vi "MPB_MAIN.vi"() -> ()   [LabVIEW 2020]
uses:
  controls/step_type.ctl
  controls/step.ctl
  controls/test results.ctl
panel:
  out "test results 2":T1
  out "test results":T1
  in  "Start Test":bool
  in  "Stop Test":bool
  in  "Exit Program":bool
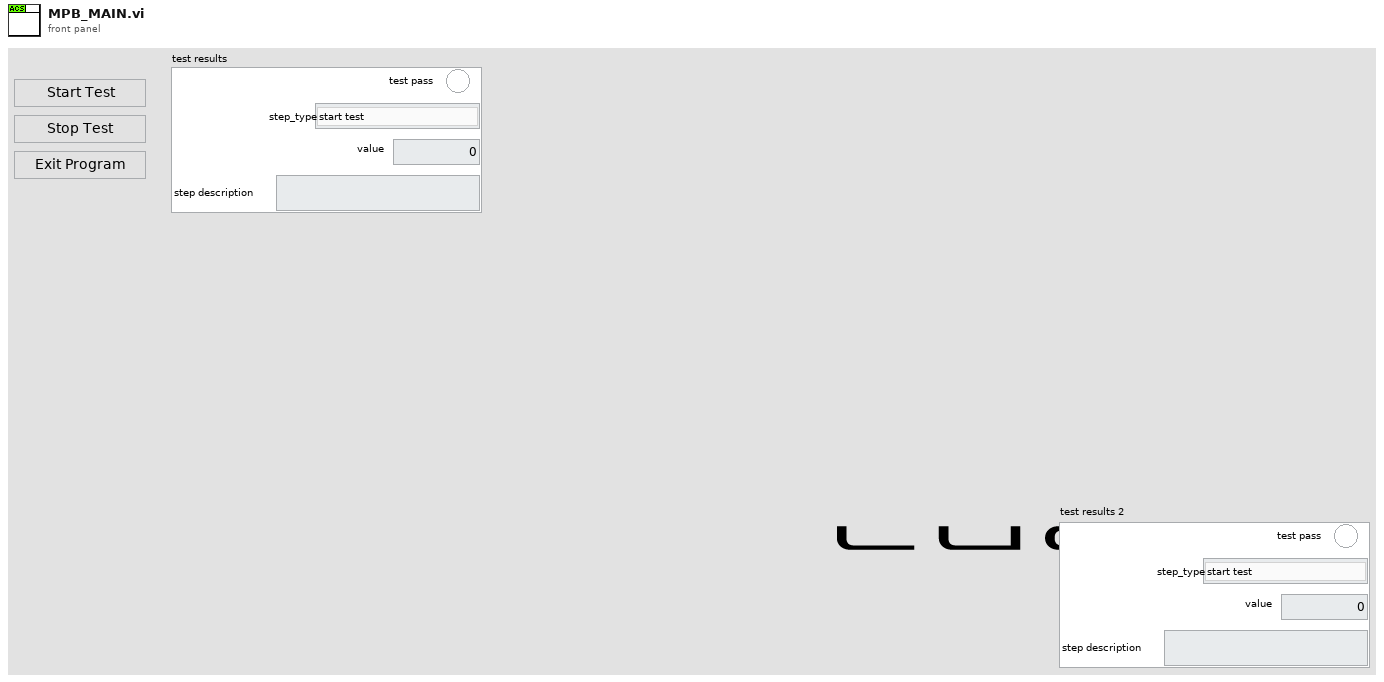
[diagram p1: front panel]
types:
  T1 = typedef "test results.ctl" = cluster{"test pass":bool, "step_type":T2, "value":dbl, "step description":string}
  T2 = typedef "step_type.ctl" = enum16{"start test", "prompt", "sequence#", "12V power supply on_off", "set_hipot_V", "set_hipot_I_limit", "set_hipot_ramping (sec)", "read_hipot_V", "read_hipot_I", "set_daq", "read_daq", "flash uds", "wait", "record_pass_fail", "error_exit"}
  T3 = typedef "step.ctl" = cluster{"VISA resource name":string, "value":dbl, "step_description (prompt)":string, "step_json":string, "save results":bool, "step_type":T2, "Step_name":string}
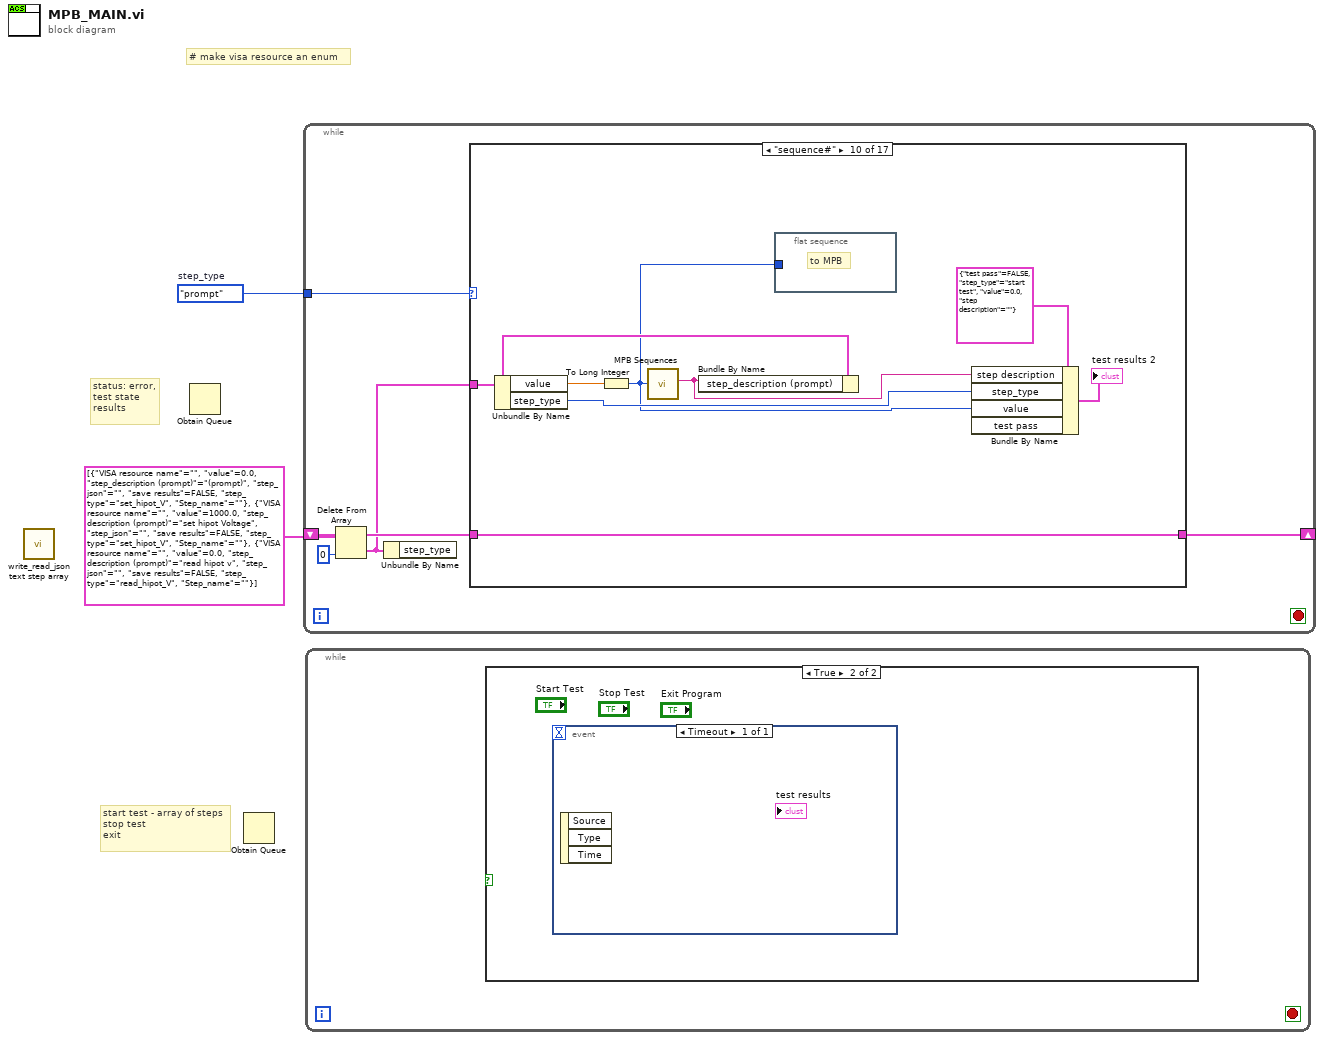
[diagram p0: block diagram]
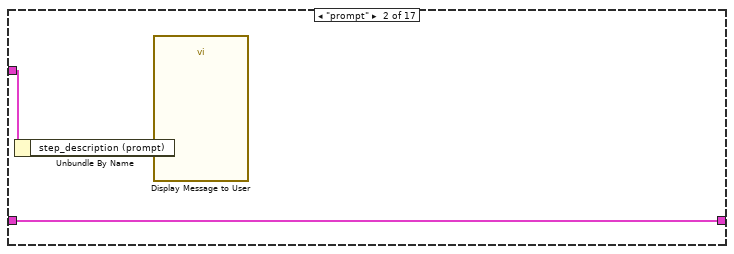
[diagram p4: hidden frame]
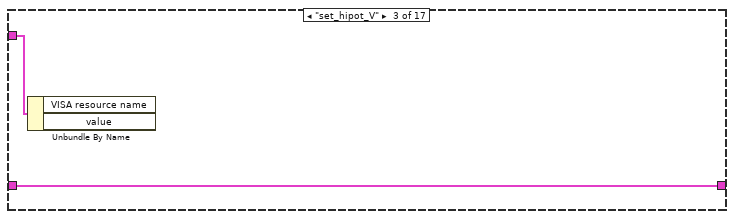
[diagram p5: hidden frame]
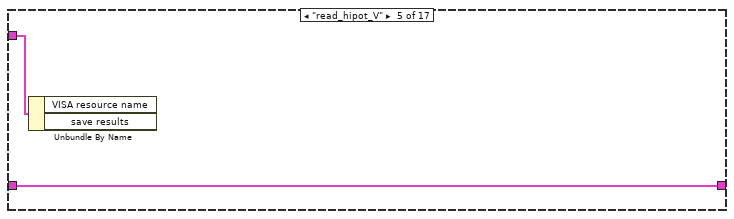
[diagram p7: hidden frame]
diagram:
  w1 = step_type."prompt"  # step_type
  # "# make visa resource an enum"
  # "start test - array of steps\nstop test\nexit"
  # "status: error,\ntest state\nresults"
  n1 = call "write_read_json text step array.vi"() -> ()  [unwired: 10 in, 2 out]
  n2 = Obtain Queue() -> ()  [unwired: 5 in, 3 out]
  n3 = Obtain Queue() -> ()  [unwired: 5 in, 3 out]
  n4 = while {
    shift-right: [w7] -> _
    shift-left: T3[] [{"VISA resource name"="", "value"=0.0, "step_description (prompt)"="(prompt)", "step_json"="", "save results"=FALSE, "step_type"=enum."set_hipot_V", "Step_name"=""}, {"VISA resource name"="", "value"=1000.0, "step_description (prompt)"="set hipot Voltage", "step_json"="", "save results"=FALSE, "step_type"=enum."set_hipot_V", "Step_name"=""}, {"VISA resource name"="", "value"=0.0, "step_description (prompt)"="read hipot v", "step_json"="", "save results"=FALSE, "step_type"=enum."read_hipot_V", "Step_name"=""}] ("json_array_from_file") -> [w9]
    tunnel: w1 -> [w3]
    stop <- _ stop-if-true
    n5 = Delete From Array(array=w9, index=0) -> (deleted portion=w5:T3, array with subset deleted=w8:T3[])  [unwired: 1 in]
    n6 = Unbundle By Name(w5) -> ("step_type"=w4:T2)
    n7 = case shown="\"sequence#\"" w3 {
      tunnel: w8 -> [w10 w13 w15 w16 w18 w19 w20 w21 w22 w30 _ _ _ _ _ _ _]
      tunnel: [w10 w13 w15 w16 w18 w19 w20 w21 w22 w30 _ _ _ _ _ _ _] -> w7
      tunnel: w5 -> [_ w12 w14 _ w17 _ _ _ _ w28 _ _ _ _ _ _ _]
      frame Default {
      }
      frame "prompt" {
        n8 = Unbundle By Name(w12) -> ("step_description (prompt)"=w11:string)
        n9 = call "Display Message to User"("Message"=w11) -> ()  [unwired: 9 in, 2 out]
      }
      frame "set_hipot_V" {
        n10 = Unbundle By Name(w14) -> ()  [unwired: 2 out]
      }
      frame "set_hipot_V" {
      }
      frame "read_hipot_V" {
        n11 = Unbundle By Name(w17) -> ()  [unwired: 2 out]
      }
      frame "read_hipot_I" {
      }
      frame "set_daq" {
      }
      frame "read_daq" {
      }
      frame "error_exit" {
      }
      frame "sequence#" {
        n12 = Unbundle By Name(w28) -> ("value"=w29:dbl, "step_type"=w24:T2)
        n13 = To Long Integer(number=w29) -> (32bit integer=w23:i32)
        n14 = call "MPB Sequences.vi"("sequence number"=w23) -> ("(description) used in test"=w25:string)  [unwired: 10 in]
        n15 = Bundle By Name(cluster=w28, "step_description (prompt)"=w25) -> ()  [unwired: 1 out]
        n16 = flat-sequence {
          tunnel: w23 -> [_]
          frame #0 {
            # "to MPB"
          }
        }
        n17 = Bundle By Name(cluster=T1 {"test pass"=FALSE, "step_type"=enum."start test", "value"=0.0, "step description"=""} ("test results 3"), "step description"=w25, "step_type"=w24, "value"=w23) -> (→"test results 2":T1)  [unwired: 1 in]
      }
      frame "start test" {
      }
      frame "12V power supply on_off" {
      }
      frame "set_hipot_I_limit" {
      }
      frame "set_hipot_ramping (sec)" {
      }
      frame "flash uds" {
      }
      frame "wait" {
      }
      frame "record_pass_fail" {
      }
    }
  }
  n18 = while {
    stop <- _ stop-if-true
    n19 = case shown="True" {
      selector: _ -> [_ _]
      frame False {
      }
      frame True {
        n20 = event shown="[0] Timeout" {
          selector: _ -> [_]
          dyn-events: _ -> [_]
          timeout: _ -> [_]
          event Timeout {
            n21 = event-data() -> ()  [unwired: 1 in, 3 out]
          }
        }
      }
    }
  }
